vi "Tegam4040 -- GetAttenuationMode.vi"(8 "error in (no error)":errorcluster, 11 "Instrument Session Handle In":u32 format="%x") -> (0 "error out":errorcluster, 2 "Attenuation":T1(ring), 3 "Instrument Session Handle Out (dupl)":u32 format="%x")   [LabVIEW 2010]
panel:
  out "VISA Error Code":i32 format="%x"
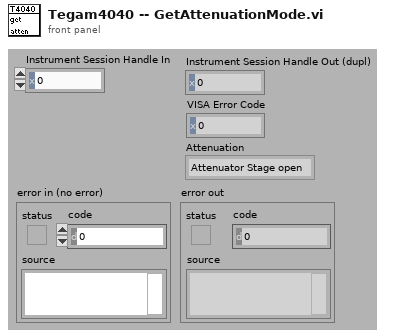
[diagram p1: front panel]
types:
  T1 = enum16{"Attenuator Stage open", "Attenuation of 1", "Attenuation of 10", "Attenuation of 100"}
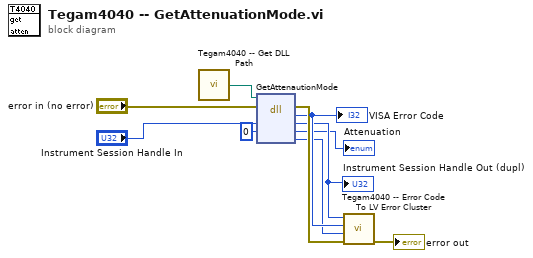
[diagram p0: block diagram]
diagram:
  n1 = call "Tegam4040 -- Get DLL Path.vi"() -> ("DLL Path"=w7:path)  [unwired: 8 in]
  n2 = dll-call lib="C:/Documents and Settings/Administrator/My Documents/Visual Studio 2005/Projects/Tegam4040CDriver/debug/Tegam4040CDriver.dll" fn="GetAttenautionMode" ("Tegam4040CDriver.dll:Close4040")(path in=w7, error in="error in (no error)", "instrSession"="Instrument Session Handle In", "inputImpedance"=u16 0) -> (error out=w9:errorcluster, "status"=w5:i32, "instrSession"=w4:u32, "inputImpedance"=→"Attenuation":u16, "driverError"=w2:i32)  [unwired: 2 in, 1 out]
  "VISA Error Code" <- w5
  "Instrument Session Handle Out (dupl)" <- w4
  n3 = call "Tegam4040 -- Error Code To LV Error Cluster.vi"("error in (no error)"=w9, "Driver Error Code"=w2, "VISA Error Code"=w5, "Instrument Session Handle"=w4) -> ("error out"=→"error out":errorcluster)  [unwired: 7 in]
